vi "Generator.vi"   [LabVIEW 2016]
uses:
  Typedefs/Generator Data Cluster.ctl
  <vilib>/Platform/TimedLoop/XDataNode/timing_clust.ctl
  <vilib>/Platform/TimedLoop/XDataNode/nitl_modes.ctl
  <vilib>/Platform/TimedLoop/XDataNode/wakeup.ctl
  <vilib>/rvi/Emulation/niFpgaSctlEmulationGetInTimedLoop.vi
  <vilib>/rvi/Emulation/niFpgaEmulationReportErrorSimple.vi
  <vilib>/rvi/Emulation/niFpgaGetClockAttributes.vi
  <vilib>/rvi/Emulation/niFpgaCriticalErrorInLSC.vi
  <vilib>/Platform/TimedLoop/XDataNode/XDataNode.xnode
  <vilib>/Platform/TimedLoop/XDataNode/XDNodeRunTimeDep.lvlib
types:
  T1 = typedef "Generator Data Cluster.ctl" = cluster{"Updated Element":u64, "Read Next?":bool, "IO Direction":u32, "IO States":u32, "Wait Ticks":u32}
  T2 = typedef "XDNodeRunTimeDep.lvlib/timing_clust.ctl" = cluster{"Expected End [f-1]":u64, "Actual End [f-1]":u64, "Finished Late? [f-1]":bool, "Expected End [i-1]":u64, "Actual End [i-1]":u64, "Finished Late? [i-1]":bool, "Expected Start [i]":u64, "Actual Start [i]":u64, "Expected Start [f]":u64, "Actual Start [f]":u64, "Source Name":string, "Structure Name":string, "Period":i64, "Deadline":i64, "Offset":i64, "Start":i64, "Priority":i32, "Timeout":i32, "Mode":T3, "Wakeup Reason":T4, "Error":errorcluster, "Source Type":string, "Secondary Source Type":string, "Global End Time":u64, "Global Start Time":u64, "Frame Duration":u64, "Iteration Duration":u64, "Assigned CPU":i32, "I/O Scan Engine Mode":u32}
  T3 = typedef "XDNodeRunTimeDep.lvlib/nitl_modes.ctl" = enum32{"No Change", "Process missed periods, maintain original phase", "Discard missed periods, maintain original phase", "Process missed periods, ignore original phase", "Discard missed periods, ignore original phase"}
  T4 = typedef "XDNodeRunTimeDep.lvlib/wakeup.ctl" = enum32{"Normal", "Aborted", "Asynchronous wakeup", "Timing source error", "Timed loop error", "Timeout"}
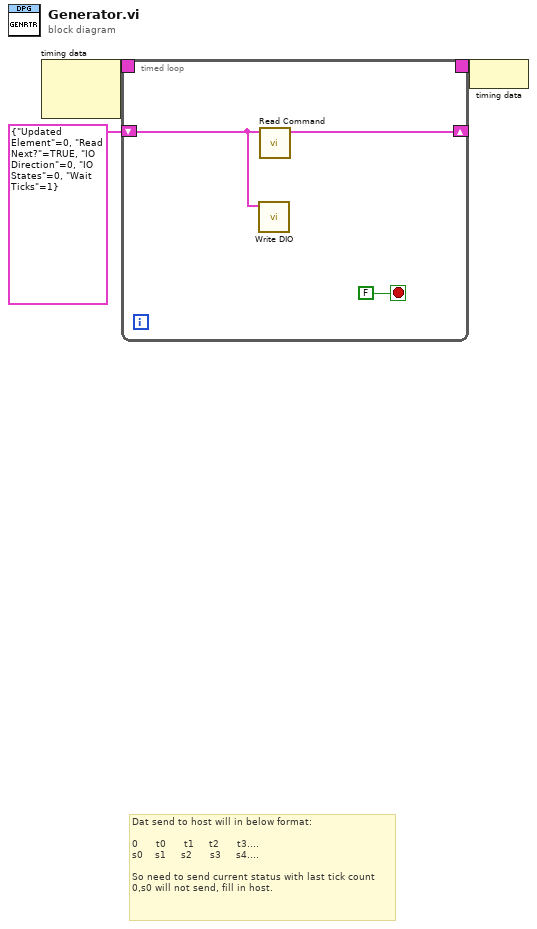
[diagram p0: block diagram]
diagram:
  # "Dat send to host will in below format:\n\n0\t     t0\t     t1\t    t2\t\t    t3....\ns0\t   s1\t    s2\t     s3\t    s4....\n\nSo need to send current status with last tick count\n0,s0 will not send, fill in host."
  n1 = node-c288() -> (w3:T2)  [unwired: 2 in]
  n2 = timed-loop {
    timing: w3 -> [_]
    timing-out: [_] -> w2
    shift-right: [w5] -> _
    shift-left: T1 {"Updated Element"=0, "Read Next?"=TRUE, "IO Direction"=0, "IO States"=0, "Wait Ticks"=1} ("Generator Data out") -> [w4]
    stop <- FALSE stop-if-true
    n3 = call "Write DIO.vi"("Generator Data in"=w4) -> ()  [unwired: 11 in]
    n4 = call "Read Command.vi"("Generator Data in"=w4) -> ("Generator Data out"=w5:T1)  [unwired: 10 in]
  }
  n5 = node-c288(w2) -> ()
